vi "Find Window Bounds.vi"() -> ()   [LabVIEW 2019]
uses:
  <vilib>/Utility/miscctls.llb/LVRectTypeDef.ctl
panel:
  in  "vi path":path
  out "Front Panel Window:Window Bounds":T1
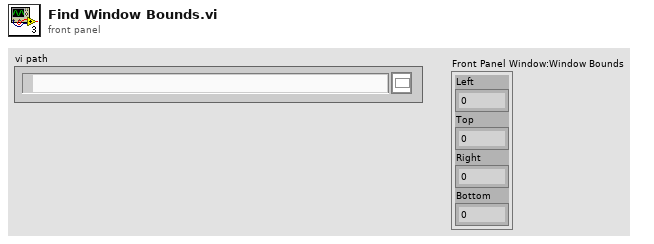
[diagram p1: front panel]
types:
  T1 = typedef "LVRectTypeDef.ctl" = cluster{"Left":i16, "Top":i16, "Right":i16, "Bottom":i16}
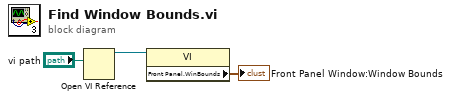
[diagram p0: block diagram]
diagram:
  n1 = Open VI Reference(vi path="vi path") -> (vi reference=w3:refnum<vi>)  [unwired: 5 in, 1 out]
  n2 = property class="VI"(reference=w3) -> ("Front Panel.WinBounds"=→"Front Panel Window:Window Bounds":T1)  [unwired: 1 in, 2 out]
